vi "(SubVI) PSD Lorentz Fit_YCC.vi"(4 "termination":cluster{"max iteration":i32, "tolerance":dbl}={"max iteration"=2000, "tolerance"=1e-15}, 5 "initial parameters":dbl[](array[numeric])=[0.05, 600.0], 6 "Frequency (Hz)":dbl[](array[numeric]), 7 "PSD (Vrms^2)":dbl[](array[numeric])) -> (1 "best fit parameters":dbl[](array[numeric]), 3 "best nonlinear fit PSD":dbl[](array[numeric]))   [LabVIEW 2014]
uses:
  <vilib>/gmath/NumericalOptimization/Nonlinear Curve Fit LM formula string.vi
  <vilib>/gmath/NI_Gmath.lvlib
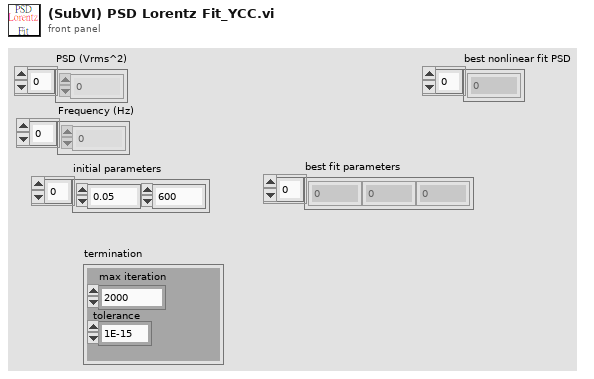
[diagram p1: front panel]
types:
  T1 = cluster{"model":string, "Parameters":string[], "x":string}
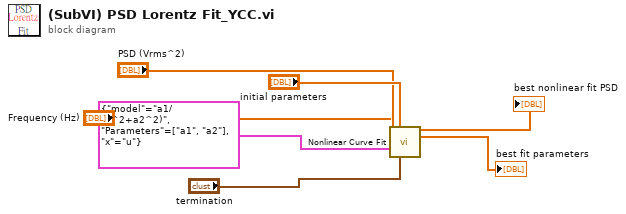
[diagram p0: block diagram]
diagram:
  n1 = call-poly <vilib>:"Nonlinear Curve Fit.vi"("Y"="PSD (Vrms^2)", "initial parameters"="initial parameters", "X"="Frequency (Hz)", "model description"=T1 {"model"="a1/(u^2+a2^2)", "Parameters"=["a1", "a2"], "x"="u"}, "termination"="termination") -> ("best nonlinear fit"=→"best nonlinear fit PSD":dbl[], "best fit parameters"=→"best fit parameters":dbl[])  [unwired: 6 in, 3 out]
